vi "sgcd4-demo-minimal.vi"() -> ()   [LabVIEW 2014]
uses:
  protocol/modbus/ni_modbus_api/API/Wrapper/Create Serial Master.vi
  protocol/modbus/ni_modbus_api/API/Master/Modbus Master.lvclass
  protocol/modbus/ni_modbus_api/API/Wrapper/API Main.lvlib
panel:
  in  "tab control":T1(tab)
  in  "range_sel":u16(ring) caption="Range Selection" items=["900 [pA]", "80 [nA]", "8 [uA]", "<not available>"]
  in  "Port":refnum<visa-resource-name>
  out "DPU_DATA":T2 caption="Latest Sensor Reading" {"REL_TREND" format="%#_5e"; "REL_LEVEL" format="%+.5f"; "RAD" format="%+#_g"}
  out "chart":sgl(graph)
  in  "stop":bool
  in  "start":bool
  out "value":sgl caption="Photocurrent" format="%_5pA"
  out "DPU_ID":T3={"HW_REV"=256, "FW_REV"=256, "NODE_SN"=256, "NODE_ADDR"=256, "NODE_TYPE"="product-name", "NODE_NAME"="node-name", "NODE_VEND"="", "RANGE_SEL"=0} caption="Sensor Description" {"RANGE_SEL" format="%0d"; "HW_REV" format="%04x"; "FW_REV" format="%04x"; "NODE_ADDR" format="%x"}
  out "DPU_CFG":T4 caption="Sensor Configuration" {"CAL_DATE" format="%08d"}
  out "elements":cluster{ext, sgl}[](array[cluster]) caption="Colelcted Data" {"?" format="%<%Y-%m-%d %H:%M:%S%2u>T"; "?" format="%#_6p"}
  out "# elements in queue":i32 caption="Number of Readings"
  out "error out":errorcluster
  in  "error in":errorcluster
  # "Select correct port,\nthen press START"
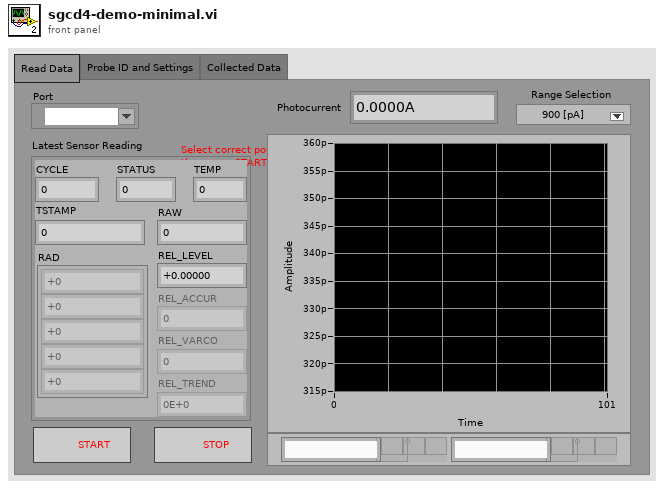
[diagram p1: front panel]
types:
  T1 = enum32{"Read Data", "Probe ID and Settings", "Collected Data"}
  T2 = cluster{"RAW":i32, "CYCLE":u16, "STATUS":u16, "TSTAMP":u32, "RAD":sgl[], "TEMP":sgl, "REL_LEVEL":sgl, "REL_ACCUR":sgl, "REL_VARCO":sgl, "REL_TREND":sgl}
  T3 = cluster{"HW_REV":u16, "FW_REV":u16, "NODE_SN":u32, "NODE_ADDR":u16, "NODE_TYPE":string, "NODE_NAME":string, "NODE_VEND":string, "RANGE_SEL":u16}
  T4 = cluster{"CAL_FACTOR":sgl[], "CAL_DATE":u32, "CAL_NAME":string[]}
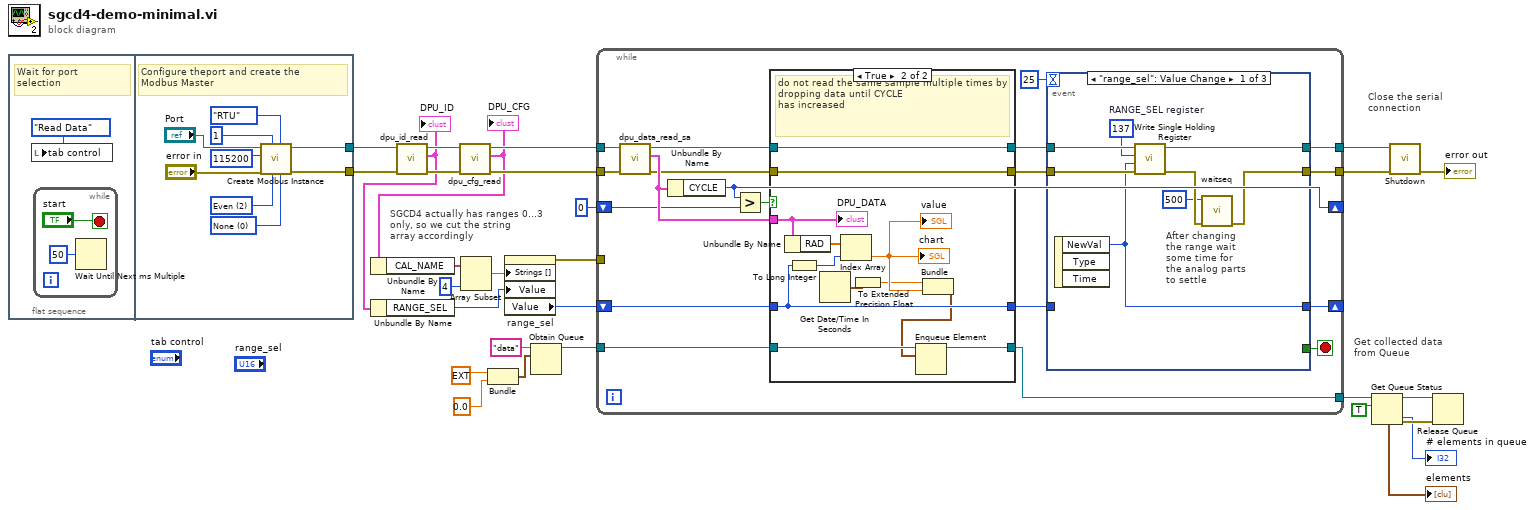
[diagram p0: block diagram]
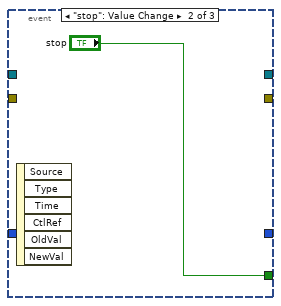
[diagram p2: hidden frame]
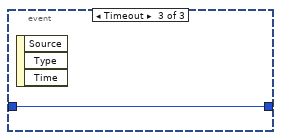
[diagram p3: hidden frame]
diagram:
  # "Close the serial\nconnection"
  # "Get collected data\nfrom Queue"
  # "SGCD4 actually has ranges 0...3\nonly, so we cut the string\narray accordingly"
  n1 = flat-sequence {
    tunnel: [w34] -> w26
    tunnel: [w33] -> w23
    frame #0 {
      # "Wait for port\nselection"
      n2 = local write "tab control"(enum32{"Read Data", "Probe ID and Settings"}."Read Data" ("tab control")) -> ()
      n3 = while {
        stop <- "start" stop-if-true
        n4 = Wait Until Next ms Multiple(millisecond multiple=u32 50) -> ()  [unwired: 1 out]
      }
    }
    frame #1 {
      w36 = u16 0 items=["None", "XON/XOFF", "RTS/CTS", "XON/XOFF & RTS/CTS", "DTR/DSR", "XON/XOFF & DTR/DSR"] ("flow control (none)")
      w37 = u16 2 items=["None", "Odd", "Even", "Mark", "Space"] ("parity (even)")
      # "Configure theport and create the\nModbus Master"
      n5 = call-poly "Create Modbus Instance.vi"("flow control (none)"=w36, "serial type"=enum16{"RTU", "ASCII"}."RTU", "parity (even)"=w37, "unit ID"=u8 1, "error in"="error in", "baud rate"=u32 115200, "VISA resource name"="Port") -> ("error out"=w33:errorcluster, "serial master instance"=w34:refnum<class "Modbus Master.lvclass">)  [unwired: 3 in]
    }
  }
  n6 = call "dpu_id_read.vi"("error in"=w23, "master"=w26) -> ("error out"=w22:errorcluster, "DPU_ID"=w19:T3, "master out"=w25:refnum<class "Modbus Master.lvclass">)  [unwired: 7 in]
  "DPU_ID" <- w19
  n7 = Unbundle By Name(w19) -> ("RANGE_SEL"=w18:u16)
  n8 = call "dpu_cfg_read.vi"("error in"=w22, "master"=w25) -> ("error out"=w21:errorcluster, "DPU_CFG"=w20:T4, "master"=w24:refnum<class "Modbus Master.lvclass">)  [unwired: 7 in]
  "DPU_CFG" <- w20
  n9 = Unbundle By Name(w20) -> ("CAL_NAME"=w15:string[])
  n10 = Array Subset(array=w15, length=4) -> (w13:string[])  [unwired: 1 in]
  n11 = Bundle(ext 0.0, sgl 0.0) -> (w4:cluster{ext, sgl})  [unwired: 1 in]
  n12 = property on="range_sel" class="Ring (strict)"("Strings []"=w13, "Value"=w18) -> (error out=w17:errorcluster, "Value"=w12:u16)  [unwired: 2 in, 1 out]
  n13 = Obtain Queue(name (unnamed)="data", element data type=w4) -> (queue out=w11:refnum<queue>)  [unwired: 3 in, 2 out]
  n14 = while {
    tunnel: w21 -> [w57]
    tunnel: w24 -> [w60]
    tunnel: [w49] -> w29
    tunnel: [w47] -> w27
    shift-right: [w54] -> _
    shift-left: u16 0 ("CYCLE") -> [w55]
    shift-right: [w46] -> _
    shift-left: w12 -> [w56]
    tunnel: w17 -> [_]
    tunnel: w11 -> [w43]
    tunnel: [w42] -> w10
    stop <- w44 stop-if-true
    n15 = call "dpu_data_read_sa.vi"("error in"=w57, "master"=w60) -> ("error out"=w52:errorcluster, "DPU_DATA"=w58:T2, "master"=w53:refnum<class "Modbus Master.lvclass">)  [unwired: 6 in, 1 out]
    n16 = Unbundle By Name(w58) -> ("CYCLE"=w54:u16)
    n17 = Greater?(x=w54, y=w55) -> (0:w59:bool)
    n18 = case shown="True" w59 {
      tunnel: w58 -> [_ w86]
      tunnel: w56 -> [w74 w83]
      tunnel: [w74 w83] -> w45
      tunnel: w53 -> [w73 w82]
      tunnel: w52 -> [w72 w81]
      tunnel: [w73 w82] -> w50
      tunnel: [w72 w81] -> w48
      tunnel: w43 -> [w71 w80]
      tunnel: [w71 w77] -> w42
      frame False {
      }
      frame True {
        # "do not read the same sample multiple times by dropping data until CYCLE\nhas increased"
        n19 = Unbundle By Name(w86) -> ("RAD"=w85:sgl[])
        n20 = To Long Integer(number=w83) -> (32bit integer=w84:i32)
        n21 = Get Date/Time In Seconds() -> (seconds since 1Jan1904=w79:timestamp)
        n22 = Index Array(array=w85, index=w84) -> (element=w78:sgl)
        "chart" <- w78
        "value" <- w78
        n23 = To Extended Precision Float(1:w79) -> (0:w75:ext)
        n24 = Bundle(w75, "Numeric"=w78) -> (w76:cluster{ext, "Numeric":sgl})  [unwired: 1 in]
        n25 = Enqueue Element(queue=w80, element=w76) -> (queue out=w77:refnum<queue>)  [unwired: 2 in, 2 out]
        "DPU_DATA" <- w86
      }
    }
    n26 = event shown="[0] \"range_sel\": Value Change" {
      selector: _ -> [_ _ _]
      dyn-events: _ -> [_ _ _]
      timeout: 25 -> [_ _ _]
      tunnel: [w66 _ _] -> w49
      tunnel: w50 -> [w68 _ _]
      tunnel: w48 -> [w67 _ _]
      tunnel: [w62 _ _] -> w47
      tunnel: [w64 _ w70] -> w46
      tunnel: w45 -> [_ _ w70]
      tunnel: [_ "stop" _] -> w44
      event "range_sel": Value Change {
        w65 = u16 137  # RANGE_SEL register
        # "After changing\nthe range wait\nsome time for\nthe analog parts\nto settle"
        n27 = event-data() -> ("NewVal"=w64:u16)  [unwired: 1 in, 2 out]
        n28 = call-dynamic "Write Single Holding Register.vi"("error in"=w67, "register to write"=w64, "address"=w65, "Modbus master in"=w68) -> ("error out"=w63:errorcluster, "Modbus master out"=w66:refnum<class "Modbus Master.lvclass">)  [unwired: 6 in]
        n29 = call "waitseq.vi"("error in"=w63, "time (ms)"=u32 500) -> ("error out"=w62:errorcluster)  [unwired: 7 in, 2 out]
      }
      event "stop": Value Change {
        n30 = event-data() -> ()  [unwired: 1 in, 6 out]
      }
      event Timeout {
        n31 = event-data() -> ()  [unwired: 1 in, 3 out]
      }
    }
  }
  n32 = Get Queue Status(queue=w10, return elements? (F)=TRUE) -> (queue out=w8:refnum<queue>, error out=w9:errorcluster, # elements in queue=→"# elements in queue":i32, elements=→"elements":cluster{ext, sgl}[])  [unwired: 1 in, 4 out]
  n33 = call-dynamic "Shutdown.vi"("error in"=w27, "Modbus master in"=w29) -> ("error out"=→"error out":errorcluster)  [unwired: 9 in]
  n34 = Release Queue(queue=w8, error in (no error)=w9) -> ()  [unwired: 1 in, 3 out]
